vi "Get Triggers Execution Time.vi"(8 "error in":errorcluster, 11 "custom device":T1 format="%.0x") -> (0 "error out":errorcluster, 2 "triggers execution time":T1 format="%.0x", 3 "custom device out":T1 format="%.0x")   [LabVIEW 2020, in "AIM MIL-STD-1553 Scripting.lvlib"]
uses:
  AIM MIL-STD-1553 Scripting.lvlib
  <vilib>/NI VeriStand/Custom Device API/Custom Device Item Ref.ctl
  Constants.vi
  <vilib>/NI VeriStand/Custom Device Tools/Custom Device Utility Library/NI VeriStand - Search for Item by Name.vi
  <vilib>/NI VeriStand/Custom Device Tools/Custom Device Utility Library/Custom Device Utility Library.lvlib
  <vilib>/NI VeriStand/Custom Device API/Custom Device API.lvlib
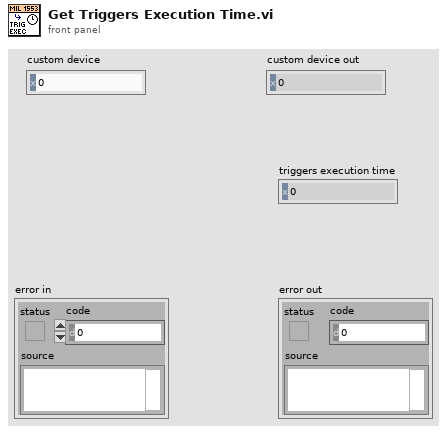
[diagram p1: front panel]
types:
  T1 = typedef "Custom Device API.lvlib/Custom Device Item Ref.ctl" = u64
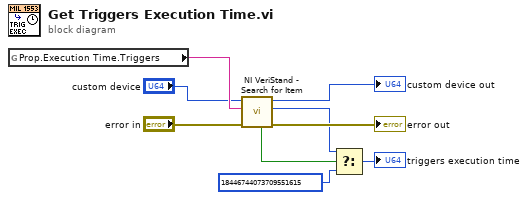
[diagram p0: block diagram]
diagram:
  n1 = global read "Constants.vi" "Prop.Execution Time.Triggers"() -> (w9:string)
  n2 = call-poly <vilib>:"NI VeriStand - Search for Item.vi"("error in"="error in", "Item Name"=w9, "Section Ref in"="custom device") -> ("error out"=→"error out":errorcluster, "Item Ref"=w4:T1, "Section Ref out"=→"custom device out":T1, "Found"=w2:bool)  [unwired: 5 in]
  n3 = Select(t=w4, s=w2, f=T1 18446744073709551615) -> (s? t:f=→"triggers execution time":T1)
